vi "Create TCP.vi"(8 "error in (no error)":errorcluster, 9 "Port":u16, 10 "Interface Address":string) -> (0 "error out":errorcluster, 3 "LINX Server out":refnum<class "LINX Server.lvclass">)   [LabVIEW 2020, in "LINX Server.lvclass"]
uses:
  LINX Server.lvclass
  LINX Base.lvclass
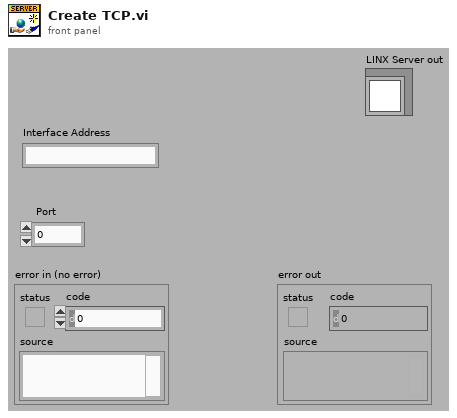
[diagram p1: front panel]
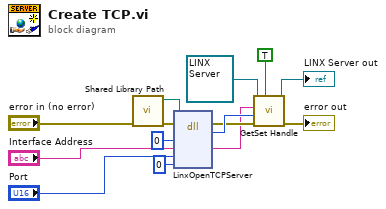
[diagram p0: block diagram]
diagram:
  n1 = call "Shared Library Path.vi"("error in (no error)"="error in (no error)") -> ("error out"=w14:errorcluster, "Path"=w12:path)  [unwired: 9 out]
  n2 = dll-call lib="Z:/Development/LabVIEW Hobbyist Toolkit/LabVIEW/vi.lib/MakerHub/LINX/Resources/libLinxDevice.dll" fn="LinxOpenTCPServer"(path in=w12, error in=w14, "LinxDevice"=u64 0, "address"="Interface Address", "port"="Port", "autolaunch"=0) -> (error out=w6:errorcluster, "LinxListener"=w7:u64, "address"=w1:string)  [unwired: 3 in, 2 out]
  n3 = call-dynamic "GetSet Handle.vi"("store (F)"=TRUE, "error in"=w6, "handle in"=w7, "connection"=w1, "LINX Base in"=refnum<class "LINX Server.lvclass"> refnum ("LINX Server out")) -> ("error out"=→"error out":errorcluster, "LINX Base out"=→"LINX Server out":refnum<class "LINX Server.lvclass">)  [unwired: 5 out]
